vi "TCPReadStrWithLength.vi"(8 "error in (no error)":errorcluster, 9 "timeout ms (25000)":i32=25000, 10 "command":string, 11 "connection ID":refnum<k5>) -> (0 "error out":errorcluster, 2 "TCP String":string, 3 "connection ID out":refnum<k5>)   [LabVIEW 2013]
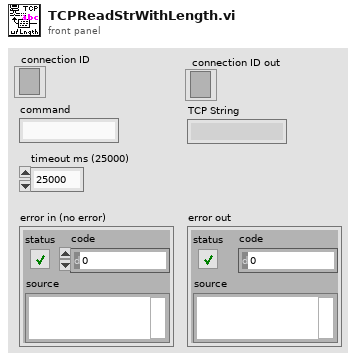
[diagram p1: front panel]
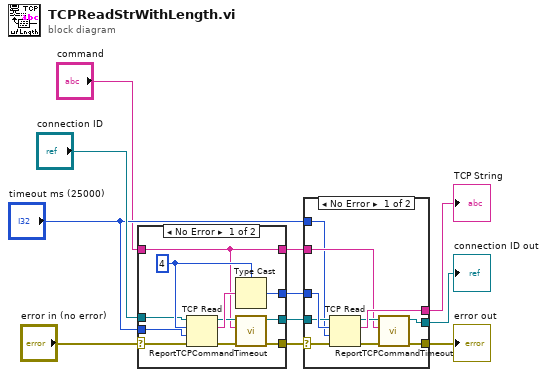
[diagram p0: block diagram]
diagram:
  n1 = case shown="No Error" "error in (no error)" {
    selector: "error in (no error)" -> [w13 w25]
    tunnel: [w21 _] -> w11
    tunnel: [w17 w24] -> w10
    tunnel: "connection ID" -> [w16 w24]
    tunnel: [w12 w23] -> w5
    tunnel: "timeout ms (25000)" -> [w15 _]
    tunnel: [w14 w25] -> w3
    tunnel: "command" -> [w12 w23]
    frame No Error {
      w20 = 4 ("bytes to read")
      n2 = TCP Read(connection ID=w16, bytes to read=w20, error in (no error)=w13, 9:w15) -> (connection ID out=w18:refnum<k5>, data out=w22:string, error out=w19:errorcluster)  [unwired: 1 in]
      n3 = Type Cast(type=w20, x=w22) -> (*(type *) &x=w21:i32)
      n4 = call "ReportTCPCommandTimeout.vi"("error in (no error)"=w19, "command"=w12, "connection ID"=w18) -> ("error out"=w14:errorcluster, "connection ID out"=w17:refnum<k5>)  [unwired: 7 in]
    }
    frame Error {
    }
  }
  n5 = case shown="No Error" w3 {
    selector: w3 -> [w26 w37]
    tunnel: w11 -> [w35 _]
    tunnel: w10 -> [w34 w36]
    tunnel: [w33 _] -> w9
    tunnel: [w30 w36] -> w7
    tunnel: [w29 w37] -> w6
    tunnel: w5 -> [w28 _]
    tunnel: "timeout ms (25000)" -> [w27 _]
    frame No Error {
      n6 = TCP Read(connection ID=w34, bytes to read=w35, error in (no error)=w26, 9:w27) -> (connection ID out=w31:refnum<k5>, data out=w33:string, error out=w32:errorcluster)  [unwired: 1 in]
      n7 = call "ReportTCPCommandTimeout.vi"("error in (no error)"=w32, "command"=w28, "connection ID"=w31) -> ("error out"=w29:errorcluster, "connection ID out"=w30:refnum<k5>)  [unwired: 7 in]
    }
    frame Error {
    }
  }
  "TCP String" <- w9
  "connection ID out" <- w7
  "error out" <- w6
